vi "BFG Ramp Data.vi"(7 "array":dbl[][](array[numeric])) -> (8 "Threshold Values":u16[](array[numeric]))   [LabVIEW 2010]
panel:
  # "•\tBattery 75% Voltage Threshold, No Load: 3.950V\n•\tBattery 75% Voltage Threshold, Stimulation On: 3.925V\n•\tBattery 50% Voltage Threshold, No Load: 3.850V\n•\tBattery 50% Voltage Threshold, Stimulation On: 3.825V\n•\tBattery 25% Voltage Threshold, No Load: 3.780V\n•\tBattery 25% Voltage Threshold, Stimulation On: 3.755V\n•\tBattery Warning Voltage Threshold, No Load: 3.740V\n•\tBattery Warning Voltage Threshold, Stimulation On: 3.715V\n•\tBattery Critical Voltage Threshold, No Load: 3.720V\n•\tBattery Critical Voltage Threshold, Stimulation On: 3.695V\n•\tMinimum Safe Stimulating Voltage, No Load: 3.700V\n•\tMinimum Safe Stimulation Voltage, Stimulation On: 3.675V\n•\tBattery Cut-off Voltage Threshold:  2.850V"
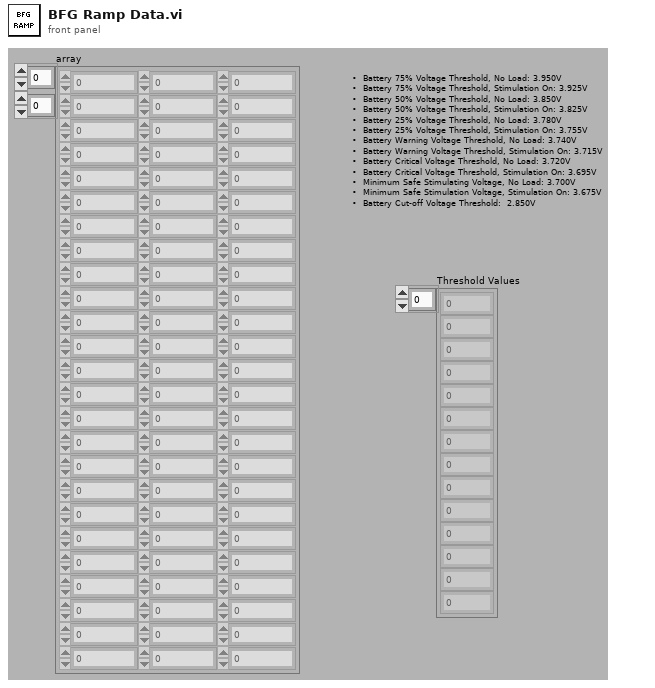
[diagram p1: front panel]
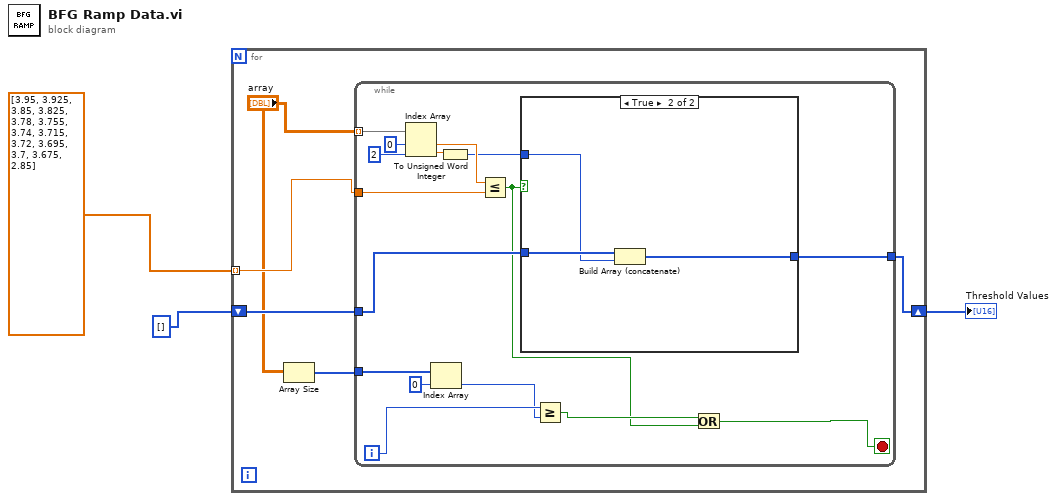
[diagram p0: block diagram]
diagram:
  n1 = for {
    tunnel: dbl[] [3.95, 3.925, 3.85, 3.825, 3.78, 3.755, 3.74, 3.715, 3.72, 3.695, 3.7, 3.675, 2.85] -> [w8] mode=indexing
    shift-right: [w6] -> w2
    shift-left: u16[] [] -> [w7]
    n2 = Array Size(array="array") -> (size(s)=w4:i32[])
    n3 = while {
      tunnel: "array" -> [w24] mode=indexing
      tunnel: w8 -> [w18]
      tunnel: w7 -> [w17]
      tunnel: [w16] -> w6
      tunnel: w4 -> [w15]
      i -> [w10]
      stop <- w11 stop-if-true
      n4 = Index Array(array=w24, index #1=0 ("index"), index #2=2 ("index")) -> (element #1=w20:dbl, element #2=w21:dbl)
      n5 = Index Array(array=w15, index=0) -> (element=w9:i32)
      n6 = To Unsigned Word Integer(number=w21) -> (unsigned 16bit integer=w19:u16)
      n7 = Less Or Equal?(x=w20, y=w18) -> (x <= y?=w12:bool)
      n8 = case shown="True" w12 {
        tunnel: w19 -> [_ w26]
        tunnel: w17 -> [w25 w28]
        tunnel: [w25 w27] -> w16
        frame False {
        }
        frame True {
          n9 = Build Array (concatenate)(w28, w26) -> (w27:u16[])
        }
      }
      n10 = Greater Or Equal?(x=w10, y=w9) -> (x >= y?=w13:bool)
      n11 = Or(x=w13, y=w12) -> (x .or. y?=w11:bool)
    }
  }
  "Threshold Values" <- w2
